vi "Get as LabVIEW Text.vi"(8 "error in (no error)":errorcluster, 10 "Name Array":string[](array[string]), 11 "JSON Value In":refnum<class "JSON Value.lvclass">) -> (0 "error out":errorcluster, 2 "LabVIEW Text":string, 3 "JSON Value Out":refnum<class "JSON Value.lvclass">)   [LabVIEW 2011, in "JSON Value.lvclass"]
uses:
  JSON Value.lvclass
panel:
  # "Value formated as LabVIEW text:\n-- no quotes on JSON strings\n-- LabVIEW text encoding <ToDo>\n-- no escaped characters <ToDo>"
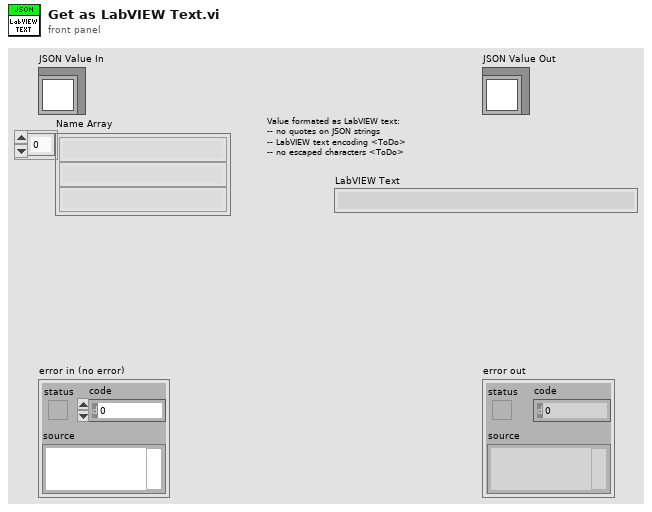
[diagram p1: front panel]
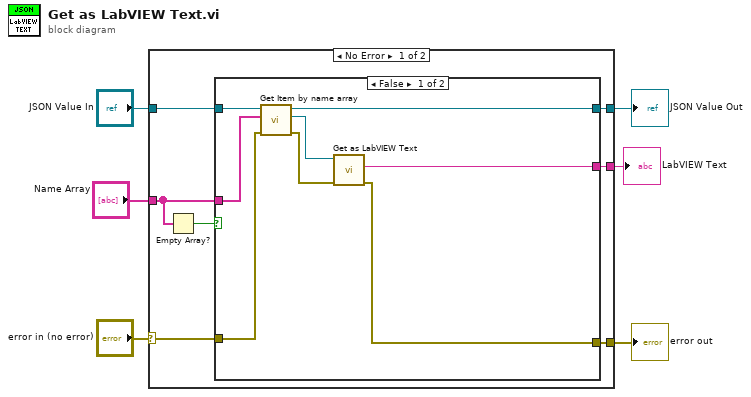
[diagram p0: block diagram]
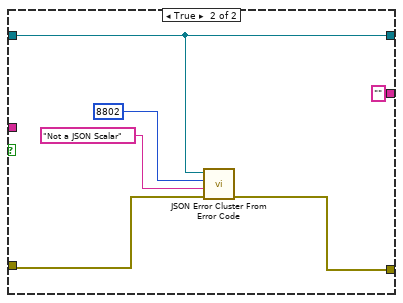
[diagram p2: hidden frame]
diagram:
  n1 = case shown="No Error" "error in (no error)" {
    selector: "error in (no error)" -> [w12 w29]
    tunnel: [w11 w29] -> w5
    tunnel: [w8 w28] -> w3
    tunnel: "JSON Value In" -> [w10 w28]
    tunnel: [w13 _] -> w2
    tunnel: "Name Array" -> [w7 _]
    frame No Error {
      n2 = Empty Array?(array=w7) -> (empty?=w9:bool)
      n3 = case shown="False" w9 {
        tunnel: [w17 ""] -> w13
        tunnel: w12 -> [w14 w24]
        tunnel: [w15 w23] -> w11
        tunnel: w10 -> [w21 w22]
        tunnel: [w19 w22] -> w8
        tunnel: w7 -> [w20 _]
        frame False {
          n4 = call "Get Item by name array.vi"("error in (no error)"=w14, "Name Array"=w20, "JSON Value In"=w21) -> ("error out"=w16:errorcluster, "Value"=w18:refnum<class "JSON Value.lvclass">, "JSON Value Out"=w19:refnum<class "JSON Value.lvclass">)  [unwired: 5 in, 1 out]
          n5 = call-dynamic "Get as LabVIEW Text.vi"("error in (no error)"=w16, "JSON Value In"=w18) -> ("error out"=w15:errorcluster, "LabVIEW Text"=w17:string)  [unwired: 7 in, 1 out]
        }
        frame True {
          n6 = call "JSON Error Cluster From Error Code.vi"("error in (no error)"=w24, "Error message"="Not a JSON Scalar", "JSON error code"=8802, "JSON Value in"=w22) -> ("error out"=w23:errorcluster)  [unwired: 6 in, 1 out]
        }
      }
    }
    frame Error {
    }
  }
  "error out" <- w5
  "JSON Value Out" <- w3
  "LabVIEW Text" <- w2
